vi "Calculate Delay.vi"(8 "error in (no error)":errorcluster, 11 "Timer in":refnum<class "Timer.lvclass">) -> (0 "error out":errorcluster, 2 "Delay":i32, 3 "Timer out":refnum<class "Timer.lvclass">)   [LabVIEW 2016, in "Timer.lvclass"]
uses:
  Timer.lvclass
  C:/Github/LabActor/Worker/Worker.lvclass
  Timer.lvclass/Timer.ctl
  Worker/Worker.lvclass/Worker.ctl
  Read Latest time.vi
  Worker/Read Cycle period.vi
  Read Start time.vi
  Write Latest time.vi
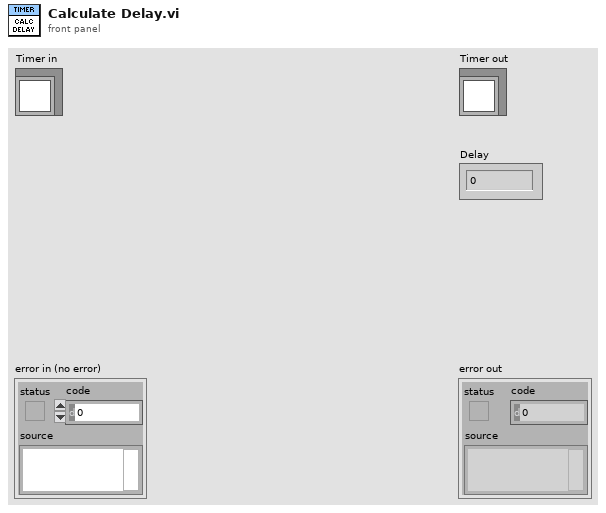
[diagram p1: front panel]
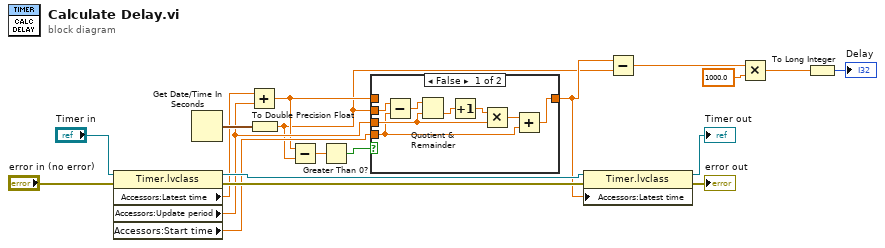
[diagram p0: block diagram]
diagram:
  n1 = property class="Timer.lvclass"(reference="Timer in", error in="error in (no error)") -> (reference out=w16:refnum<class "Timer.lvclass">, error out=w15:errorcluster, "Accessors:Latest time"=w12:dbl, "Accessors:Update period"=w10:dbl, "Accessors:Start time"=w9:dbl)
  n2 = Get Date/Time In Seconds() -> (seconds since 1Jan1904=w17:timestamp)
  n3 = Add(x=w12, y=w10) -> (x+y=w6:dbl)
  n4 = To Double Precision Float(number=w17) -> (double precision float=w2:dbl)
  n5 = Subtract(x=w6, y=w2) -> (x-y=w4:dbl)
  n6 = Greater Than 0?(x=w4) -> (x > 0?=w11:bool)
  n7 = case shown="False" w11 {
    tunnel: w2 -> [w24 _]
    tunnel: w9 -> [w20 _]
    tunnel: w10 -> [w23 _]
    tunnel: w6 -> [_ w28]
    tunnel: [w21 w28] -> w3
    frame False {
      n8 = Subtract(x=w24, y=w20) -> (x-y=w22:dbl)
      n9 = Quotient & Remainder(x=w22, y=w23) -> (floor(x/y)=w25:dbl)  [unwired: 1 out]
      n10 = Increment(x=w25) -> (x+1=w26:dbl)
      n11 = Multiply(x=w26, y=w23) -> (x*y=w27:dbl)
      n12 = Add(x=w27, y=w20) -> (x+y=w21:dbl)
    }
    frame True {
    }
  }
  n13 = property class="Timer.lvclass"(reference=w16, error in=w15, "Accessors:Latest time"=w3) -> (reference out=→"Timer out":refnum<class "Timer.lvclass">, error out=→"error out":errorcluster)
  n14 = Subtract(x=w3, y=w2) -> (x-y=w1:dbl)
  n15 = Multiply(x=w1, y=1000.0) -> (x*y=w8:dbl)
  n16 = To Long Integer(number=w8) -> (32bit integer=→"Delay":i32)
